vi "PXI-Change AO Gains (by channel, scalar).vi"(0 "Multiplier":dbl, 5 "Gain":dbl, 7 "AO Channel":u16, 11 "error in (no error)":errorcluster) -> (15 "error out":errorcluster)   [LabVIEW 2015]
doc: "This is a test."
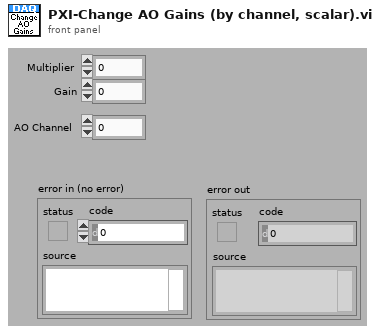
[diagram p1: front panel]
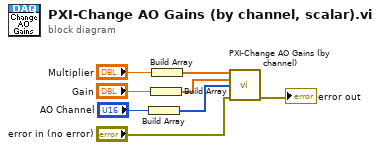
[diagram p0: block diagram]
diagram:
  n1 = Build Array("AO Channel") -> (w3:u16[])
  n2 = Build Array("Gain") -> (w4:dbl[])
  n3 = Build Array("Multiplier") -> (w5:dbl[])
  n4 = call "PXI-Change AO Gains (by channel).vi"("Multipliers"=w5, "Gains"=w4, "AO channels"=w3, "error in (no error)"="error in (no error)") -> ("error out"=→"error out":errorcluster)  [unwired: 11 in]
